vi "Release (SubVI).vi"() -> ()   [LabVIEW 2017]
uses:
  <vilib>/myRIO/Instrument Drivers/Onboard IO/Encoder/typedefs/Encoder Reference.ctl
  <vilib>/myRIO/Common/Instrument Driver Framework/Utilities/typedefs/myRIO Generic Hardware Reference.ctl
  <vilib>/myRIO/Common/Instrument Driver Framework/Utilities/typedefs/Hardware Version Enum.ctl
  <vilib>/myRIO/Common/Instrument Driver Framework/Utilities/typedefs/myRIO v1.0 Reference.ctl
  <vilib>/myRIO/Common/Instrument Driver Framework/Utilities/typedefs/Generic FPGA Reference.ctl
  <vilib>/myRIO/Common/Instrument Driver Framework/myRIO v1.0/Encoder/typedefs/Encoder Channels Enum.ctl
  <vilib>/myRIO/Instrument Drivers/Onboard IO/DIO/typedefs/DIO Reference.ctl
  <vilib>/myRIO/Common/Instrument Driver Framework/myRIO v1.0/DIO/typedefs/DIO Channels List.ctl
  <vilib>/myRIO/Common/Instrument Driver Framework/myRIO v1.0/DIO/typedefs/DIO Channels Enum.ctl
  <vilib>/userdefined/High Color/nirio_resource_hc.ctl
  <vilib>/myRIO/Common/Instrument Driver Framework/Utilities/vis/Is FPGA Ref Available.vi
  <vilib>/myRIO/Common/Instrument Driver Framework/myRIO v1.0/DIO/vis/myRIO v1.1 Open DIO.vi
  <vilib>/myRIO/Instrument Drivers/Onboard IO/DIO/vis/Write.vi
  <vilib>/myRIO/Common/Instrument Driver Framework/Utilities/vis/Validate Channels.vi
  <vilib>/myRIO/Common/Instrument Driver Framework/myRIO v1.0/DIO/vis/myRIO v1.0 Reserve DIO.vi
  <vilib>/myRIO/Common/Instrument Driver Framework/myRIO v1.0/Resource Manager/vis/myRIO v1.0 Reserve Channel List.vi
  <vilib>/myRIO/Common/Instrument Driver Framework/myRIO v1.0/DIO/vis/myRIO v1.0 Build MUX Configuration DIO.vi
  <vilib>/myRIO/Common/Instrument Driver Framework/myRIO v1.0/Resource Manager/vis/myRIO v1.0 Reserve Channel.vi
  <vilib>/myRIO/Common/Instrument Driver Framework/myRIO v1.0/Resource Manager/vis/myRIO v1.0 Unreserve Channel.vi
  <vilib>/myRIO/Common/Instrument Driver Framework/myRIO v1.0/Resource Manager/vis/myRIO v1.0 Create Configuration List.vi
  <vilib>/myRIO/Common/Instrument Driver Framework/myRIO v1.0/Resource Manager/vis/myRIO v1.0 Build Mutex Name.vi
  <vilib>/Utility/error.llb/Error Cluster From Error Code.vi
  <vilib>/myRIO/Common/Instrument Driver Framework/myRIO v1.0/Encoder/vis/myRIO v1.0 Read Encoder.vi
  <vilib>/Utility/VariantDataType/GetNumericInfo.vi
  <vilib>/myRIO/Common/Instrument Driver Framework/myRIO v1.0/myRIO v1.1 Open.vi
  <vilib>/myRIO/Common/Instrument Driver Framework/Utilities/vis/IO Manager.vi
  <vilib>/myRIO/Common/Instrument Driver Framework/Utilities/vis/Configuration Manager.vi
  <vilib>/myRIO/Common/Instrument Driver Framework/myRIO v1.0/Resource Manager/vis/myRIO v1.0 Configure IO.vi
  <vilib>/myRIO/Common/Instrument Driver Framework/myRIO v1.0/myRIO v1.0 Close.vi
  <vilib>/myRIO/Common/Instrument Driver Framework/myRIO v1.0/DIO/vis/myRIO v1.0 Write DIO.vi
  <vilib>/myRIO/Express VI/Onboard IO/DO/DO Express VI.xnode
  <vilib>/myRIO/Instrument Drivers/Onboard IO/DIO/vis/myRIO DIO Open.xnode
  <vilib>/myRIO/Instrument Drivers/Onboard IO/Encoder/Encoder.lvlib
  <vilib>/myRIO/Instrument Drivers/Onboard IO/DIO/DIO.lvlib
panel:
  in  "G_upper bound":i32
  out "G enc val":i32
  out "G+":bool
  in  "stopG":bool
  in  "G_Encoder Ref In":T1
  in  "M_Encoder Ref In":T1
  out "error out":errorcluster
  in  "error in (no error)":errorcluster
  in  "M_upper bound":i32
  out "M enc val":i32
  in  "stopM":bool
  out "M+":bool
  # "SET UP THE VALUES"
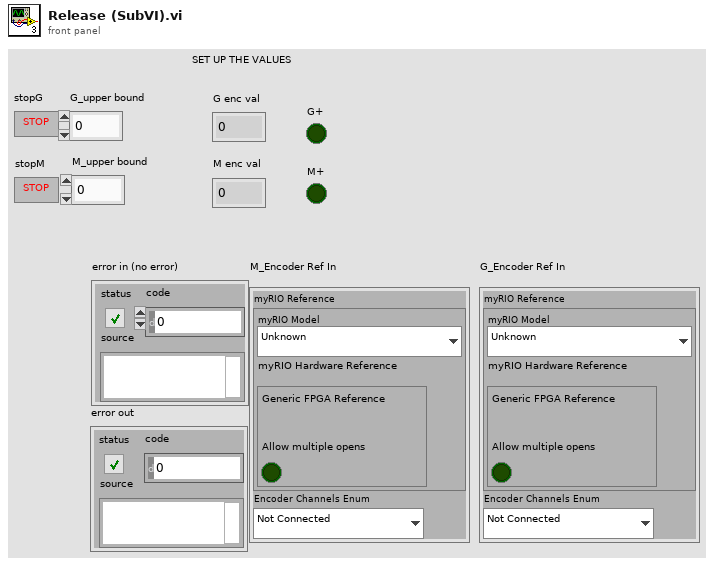
[diagram p1: front panel]
types:
  T1 = typedef "Encoder.lvlib/Encoder Reference.ctl" = cluster{"myRIO Reference":T2, "Encoder Channels Enum":T6}
  T2 = typedef "myRIO Generic Hardware Reference.ctl" = cluster{"myRIO Model":T3, "myRIO Hardware Reference":T4}
  T3 = typedef "Hardware Version Enum.ctl" = enum16{"Unknown", "myRIO-1900", "myRIO-1950", "roboRIO", "NI ELVIS RIO CM"}
  T4 = typedef "myRIO v1.0 Reference.ctl" = cluster{"Generic FPGA Reference":T5, "Allow multiple opens":bool}
  T5 = typedef "Generic FPGA Reference.ctl" = refnum<k20>
  T6 = typedef "Encoder Channels Enum.ctl" = enum16{"Not Connected", "C/ENC0", "C/ENC1", "A/ENC", "B/ENC", "DIO/ENC0", "DIO/ENC1", "DIO/ENC2", "DIO/ENC3", "DIO/ENC4"}
  T7 = typedef "DIO.lvlib/DIO Reference.ctl" = cluster{"myRIO Reference":T2, "DIO Channels List":T8}
  T8 = typedef "DIO Channels List.ctl" = T9[]
  T9 = typedef "DIO Channels Enum.ctl" = enum16{"Not Connected", "C/DIO0", "C/DIO1", "C/DIO2", "C/DIO3", "C/DIO4", "C/DIO5", "C/DIO6", "C/DIO7", "A/DIO0", "A/DIO1", "A/DIO2", "A/DIO3", "A/DIO4", "A/DIO5", "A/DIO6", "A/DIO7", "A/DIO8", "A/DIO9", "A/DIO10", "A/DIO11", "A/DIO12", "A/DIO13", "A/DIO14", "A/DIO15", "B/DIO0", "B/DIO1", "B/DIO2", "B/DIO3", "B/DIO4", "B/DIO5", "B/DIO6", "B/DIO7", "B/DIO8", "B/DIO9", "B/DIO10", "B/DIO11", "B/DIO12", "B/DIO13", "B/DIO14", "B/DIO15", "LED0", "LED1", "LED2", "LED3", "Button0", "DIO/DIO0", "DIO/DIO1", "DIO/DIO2", "DIO/DIO3", "DIO/DIO4", "DIO/DIO5", "DIO/DIO6", "DIO/DIO7", "DIO/DIO8", "DIO/DIO9", "SPI/CS0", "SPI/CS1", "SPI/CS2", "SPI/CS3", "LED RADIO (Green)", "LED RADIO (Red)", "LED COMM (Green)", "LED COMM (Red)", "LED MODE (Green)", "LED MODE (Red)"}
  T10 = typedef "nirio_resource_hc.ctl" = tag
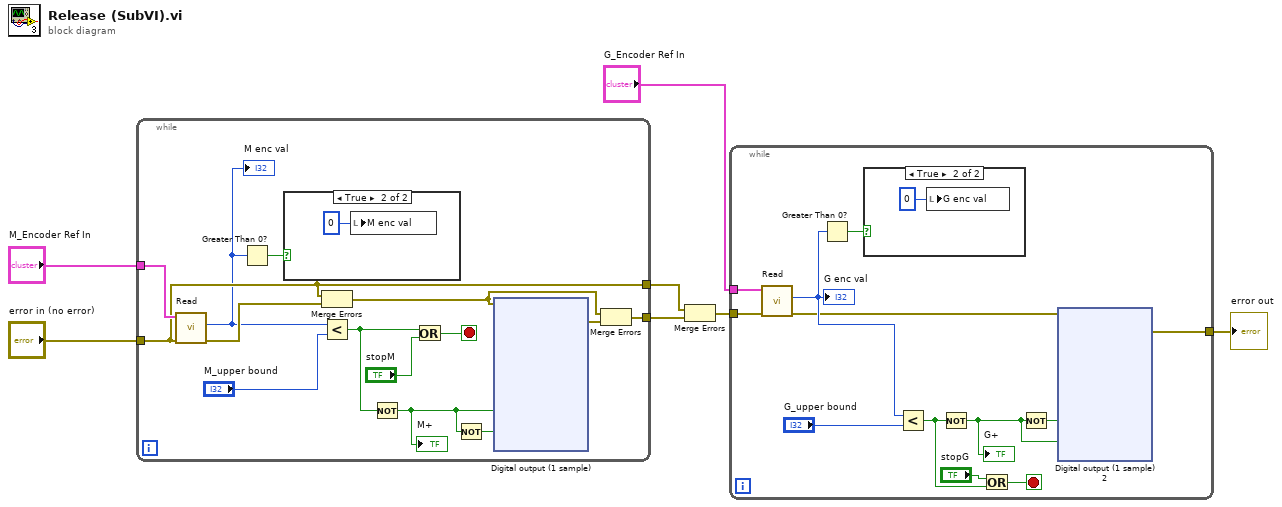
[diagram p0: block diagram]
diagram:
  n1 = while {
    tunnel: "error in (no error)" -> [w17]
    tunnel: [w17] -> w6
    tunnel: [w20] -> w5
    tunnel: "M_Encoder Ref In" -> [w18]
    stop <- w14 stop-if-true
    n2 = call <vilib>:"Read.vi"("error in (no error)"=w17, "Encoder Ref In"=w18) -> ("error out"=w16:errorcluster, "Counter Value"=w15:i32)  [unwired: 5 in, 3 out]
    "M enc val" <- w15
    n3 = Greater Than 0?(x=w15) -> (x > 0?=w8:bool)
    n4 = case shown="True" w8 {
      frame False {
      }
      frame True {
        n5 = local write "M enc val"(0 ("M enc val")) -> ()
      }
    }
    n6 = Merge Errors(w17, w16) -> (w9:errorcluster)
    n7 = Less?(x=w15, y="M_upper bound") -> (x < y?=w19:bool)
    n8 = Not(x=w19) -> (.not. x?=w11:bool)
    "M+" <- w11
    n9 = Or(x=w19, y="stopM") -> (x .or. y?=w14:bool)
    n10 = Not(x=w11) -> (.not. x?=w12:bool)
    n11 = xnode "Digital output (1 sample)"("M+ (B/DIO5 (Pin 21))"=w11, "M- (B/DIO6 (Pin 23))"=w12, "error in (no error)"=w9) -> ("error out"=w10:errorcluster)
    n12 = Merge Errors(w9, w10) -> (w20:errorcluster)
  }
  n13 = Merge Errors(w6, w5) -> (w3:errorcluster)
  n14 = while {
    tunnel: w3 -> [w66]
    tunnel: [w59] -> w2
    tunnel: "G_Encoder Ref In" -> [w65]
    stop <- w61 stop-if-true
    n15 = call <vilib>:"Read.vi"("error in (no error)"=w66, "Encoder Ref In"=w65) -> ("error out"=w67:errorcluster, "Counter Value"=w69:i32)  [unwired: 5 in, 3 out]
    "G enc val" <- w69
    n16 = Greater Than 0?(x=w69) -> (x > 0?=w68:bool)
    n17 = case shown="True" w68 {
      frame False {
      }
      frame True {
        n18 = local write "G enc val"(0 ("Value")) -> ()
      }
    }
    n19 = Less?(x=w69, y="G_upper bound") -> (x < y?=w60:bool)
    n20 = Not(x=w60) -> (.not. x?=w64:bool)
    "G+" <- w64
    n21 = Or(x="stopG", y=w60) -> (x .or. y?=w61:bool)
    n22 = Not(x=w64) -> (.not. x?=w63:bool)
    n23 = xnode "Digital output (1 sample) 2"("G- (B/DIO7 (Pin 25))"=w63, "G+ (B/DIO13 (Pin 26))"=w64, "error in (no error)"=w67) -> ("error out"=w59:errorcluster)
  }
  "error out" <- w2
